vi "Lookup Config Child.vi"(8 "error in (no error)":errorcluster, 10 "Name":string, 11 "Module in":refnum<class "Module.lvclass">) -> (0 "error out":errorcluster, 1 "Found":bool, 2 "Config Child":refnum<class "Config Element.lvclass">, 3 "Module out":refnum<class "Module.lvclass">)   [LabVIEW 2020, in "Volatus.lvlib" / "Module.lvclass"]
uses:
  Module.lvclass
  Module.lvclass/Module.ctl
  VolatusConfig/VolatusConfigElement/VolatusConfigElement.lvclass
  lv-cdm/CDM-Config/Config Element/Config Element.lvclass
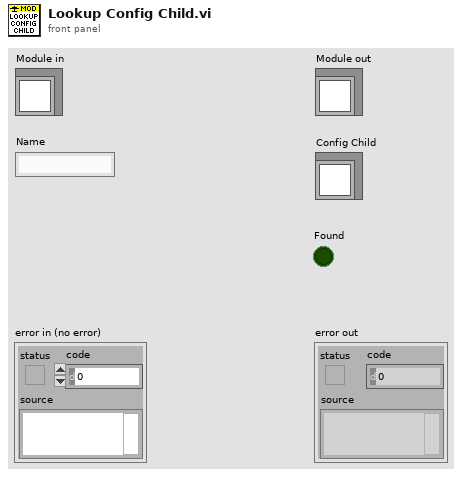
[diagram p1: front panel]
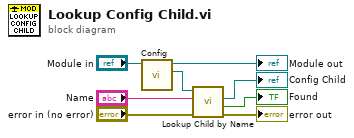
[diagram p0: block diagram]
diagram:
  n1 = call "Config.vi"("Module in"="Module in") -> ("Config"=w6:refnum<class "VolatusConfigElement.lvclass">, "Module out"=→"Module out":refnum<class "Module.lvclass">)  [unwired: 9 in]
  n2 = call "Lookup Child by Name.vi"("error in (no error)"="error in (no error)", "Child Name"="Name", "VolatusConfigElement in"=w6) -> ("error out"=→"error out":errorcluster, "Found"=→"Found":bool, "Child"=→"Config Child":refnum<class "Config Element.lvclass">)  [unwired: 5 in, 1 out]
